vi "3.2.0 Kalman Main.vi"(1 "State Variable X":T1, 6 "Covariance P":T1) -> (0 "State Vector X":T2, 2 "Control Input Model B":T1, 3 "Real Matrix":T1, 4 "Multiply Error":i32, 5 "State Update Matrix F":T1, 7 "Covariance P 2":T1, 8 "Hk-Observation Matrix":dbl[][](array[numeric])=[[0.0, 0.0, 0.0, 1.0, 0.0, 0.0], [0.0, 0.0, 0.0, 0.0, 1.0, 0.0], [0.0, 0.0, 0.0, 0.0, 0.0, 1.0]])   [LabVIEW 2010]
uses:
  <vilib>/Analysis/Matrix/Datatypes/RealMatrix.ctl
  4-High Neurons/4.2/4.2.0 Kalman State.ctl
  <vilib>/Analysis/baseanly.llb/Real A x B.vi
  <vilib>/Analysis/NI_AALBase.lvlib
  <vilib>/Analysis/Matrix/NI_Matrix.lvlib
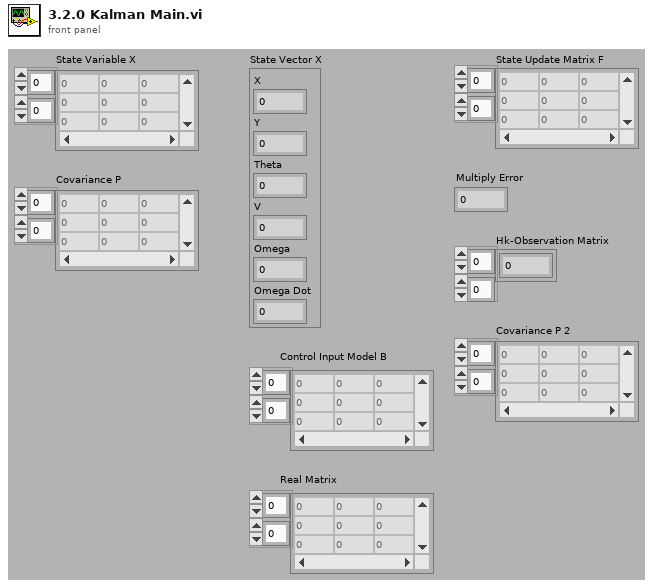
[diagram p1: front panel]
types:
  T1 = typedef "NI_Matrix.lvlib/RealMatrix.ctl" = dbl[][]
  T2 = typedef "4.2.0 Kalman State.ctl" = cluster{"X":dbl, "Y":dbl, "Theta":dbl, "V":dbl, "Omega":dbl, "Omega Dot":dbl}
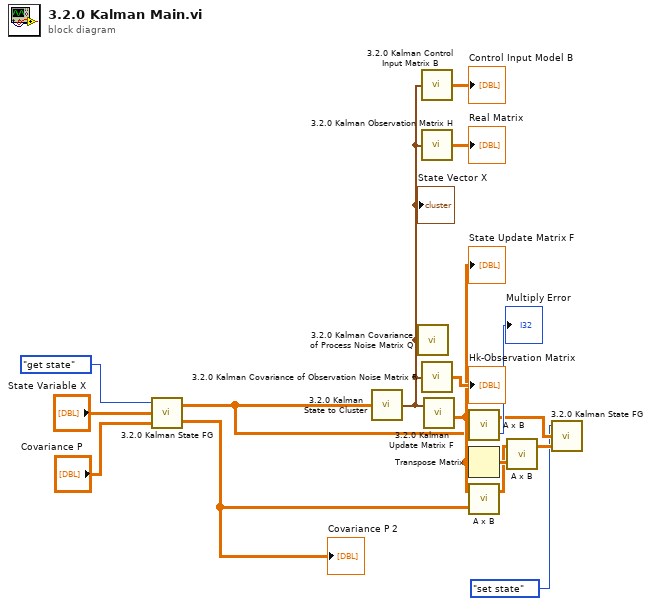
[diagram p0: block diagram]
diagram:
  n1 = call "3.2.0 Kalman State FG.vi"("Covariance P 2"="Covariance P", "State Variable X 2"="State Variable X", "Enum"=enum16{"get state", "set state"}."get state") -> ("Covariance P"=w9:T1, "State Variable X"=w5:T1)
  "Covariance P 2" <- w9
  n2 = call "3.2.0 Kalman State to Cluster.vi"("State Variable X 3"=w5) -> ("State Vector X"=w15:T2)
  "State Vector X" <- w15
  n3 = call "3.2.0 Kalman Covariance of Process Noise Matrix Q.vi"("State Vector X"=w15) -> ()  [unwired: 1 out]
  n4 = call "3.2.0 Kalman Control Input Matrix B.vi"("State Vector X"=w15) -> ("Real Matrix"=→"Control Input Model B":T1)
  n5 = call "3.2.0 Kalman Observation Matrix H.vi"("State Vector X"=w15) -> ("Real Matrix"=→"Real Matrix":T1)
  n6 = call "3.2.0 Kalman Covariance of Observation Noise Matrix R.vi"("State Vector X"=w15) -> ("Covariance of Observation Noise R"=→"Hk-Observation Matrix":dbl[][])
  n7 = call "3.2.0 Kalman Update Matrix F.vi"("State Vector X"=w15) -> ("Update Matrix F"=w8:T1)  [unwired: 4 in]
  "State Update Matrix F" <- w8
  n8 = call-poly <vilib>:"A x B.vi"("B"=w5, "A"=w8) -> ("error"=→"Multiply Error":i32, "A x B"=w6:T1)
  n9 = Transpose Matrix(1:w8) -> (0:w11:T1)
  n10 = call-poly <vilib>:"A x B.vi"("B"=w9, "A"=w8) -> ("A x B"=w10:T1)  [unwired: 1 out]
  n11 = call-poly <vilib>:"A x B.vi"("B"=w11, "A"=w10) -> ("A x B"=w12:T1)  [unwired: 1 out]
  n12 = call "3.2.0 Kalman State FG.vi"("Covariance P 2"=w12, "State Variable X 2"=w6, "Enum"=enum16{"get state", "set state"}."set state") -> ()  [unwired: 2 out]
